vi "Corridor 1 to Corridor 3.vi"(0 "Starting Position":T5=enum."Far Right", 1 "C1 to C3":T4, 3 "Command Info In":T1) -> (10 "Command Info Out":T1)   [LabVIEW 2017]
uses:
  <vilib>/Rock Robotics/WPI/Framework/Command Status Info.ctl
  <vilib>/Rock Robotics/WPI/Framework/Completion Status.ctl
  <vilib>/Rock Robotics/WPI/Framework/Completion Notifier.ctl
  Support Code/Starting Position.ctl
  Block Clusters/C1 to C3.ctl
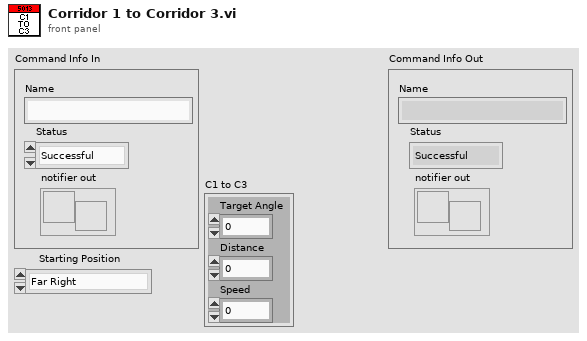
[diagram p1: front panel]
types:
  T1 = typedef "Command Status Info.ctl" = cluster{"Name":string, "Status":T2, "notifier out":T3}
  T2 = typedef "Completion Status.ctl" = enum16{"Successful", "Aborted", "Incomplete"}
  T3 = typedef "Completion Notifier.ctl" = refnum<notifier>
  T4 = typedef "C1 to C3.ctl" = cluster{"Target Angle":dbl, "Distance":dbl, "Speed":dbl}
  T5 = typedef "Starting Position.ctl" = enum16{"Far Left", "Center", "Far Right"}
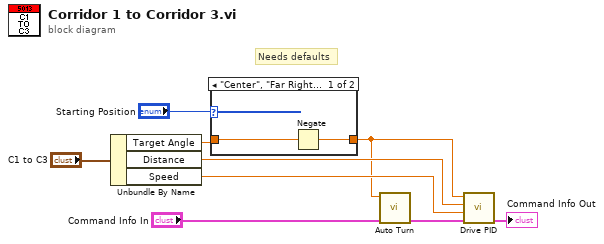
[diagram p0: block diagram]
diagram:
  # "Needs defaults"
  n1 = Unbundle By Name("C1 to C3") -> ("Target Angle"=w7:dbl, "Distance"=w6:dbl, "Speed"=w5:dbl)
  n2 = case shown="\"Center\", \"Far Right\"" "Starting Position" {
    tunnel: w7 -> [w11 w12]
    tunnel: [w10 w12] -> w2
    frame "Center", "Far Right" {
      n3 = Negate(x=w11) -> (-x=w10:dbl)
    }
    frame "Far Left", Default {
    }
  }
  n4 = call "Auto Turn.vi"("Command Info In"="Command Info In", "Target Angle"=w2) -> ("Command Info Out"=w3:T1)  [unwired: 9 in]
  n5 = call "Drive PID.vi"("Command Info In"=w3, "Speed"=w5, "Distance"=w6, "Target Angle"=w2) -> ("Command Info Out"=→"Command Info Out":T1)  [unwired: 7 in]
